vi "Substitute Actor.vi"(10 "Substitute Actor in":refnum<class "Actor.lvclass">, 11 "Current ViewableActor":refnum<class "ViewableActor.lvclass">) -> (0 "error out":errorcluster, 2 "Substitute Actor out":refnum<class "Actor.lvclass">)   [LabVIEW 2020, in "ViewableActor.lvlib" / "ViewableActor.lvclass"]
doc: "(<B>Filename</B>: Actor Framework.lvlib:Actor.lvclass:Substitute Actor.vi)\n\nThis method copies information from the <b>Current Actor</b> to the <b>Substitute Actor</b>, including the to-self and the to-caller queue references. The purpose of this function is to allow an actor to define a method that replaces itself with another actor, useful for implementing a State Pattern Actor. Child classes should override this method to copy any additional fields that they need from the current to the substitute.\n\nThis method may return error code 678010: Illegal substitution. Overrides of this method may choose to return this error if the new actor is not one that is an appropriate substitute for the current actor, for whatever standards of \"appropriate\" are chosen for the current actor. If returning an error, override VIs should return the unmodified <b>Current Actor</b> as <b>Substitute Actor out</b>."
uses:
  ViewableActor.lvclass
  C:/Program Files (x86)/National Instruments/LabVIEW 2020/vi.lib/ActorFramework/Actor/Actor.lvclass
  <vilib>/ActorFramework/Actor/Actor.lvclass
  ViewableActor.lvclass/ViewableActor.ctl
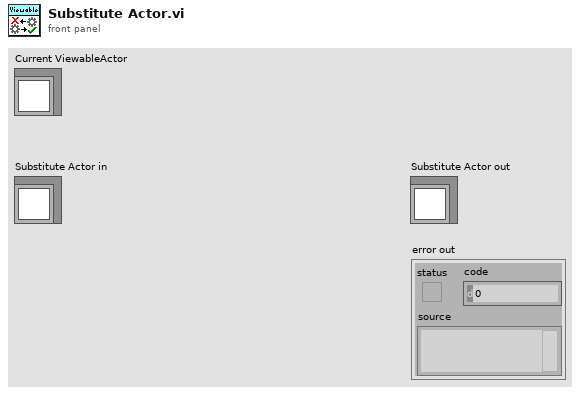
[diagram p1: front panel]
types:
  T1 = typedef "LVRectTypeDef.ctl" = cluster{"Left":i16, "Top":i16, "Right":i16, "Bottom":i16}
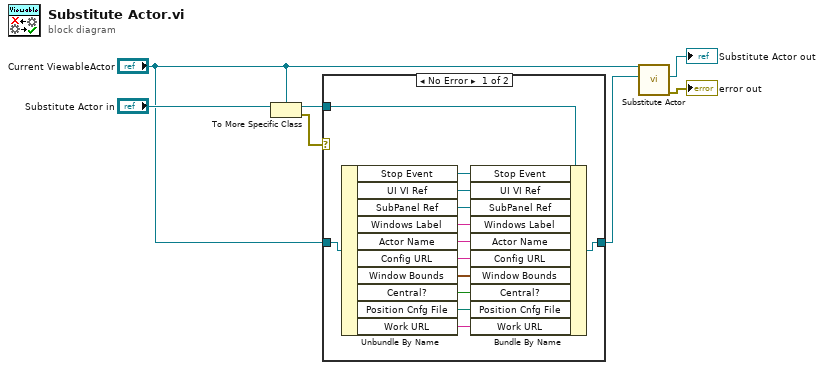
[diagram p0: block diagram]
diagram:
  n1 = To More Specific Class(target class="Current ViewableActor", reference="Substitute Actor in") -> (specific class reference=w4:refnum<class "ViewableActor.lvclass">, error out=w1:errorcluster)  [unwired: 1 in]
  n2 = case shown="No Error" w1 {
    tunnel: w4 -> [w20 _]
    tunnel: "Current ViewableActor" -> [w19 w21]
    tunnel: [w18 w21] -> w2
    frame No Error {
      n3 = Unbundle By Name(w19) -> ("Stop Event"=w17:refnum<user-event>, "UI VI Ref"=w16:refnum<vi>, "SubPanel Ref"=w15:refnum<vi>, "Windows Label"=w14:string, "Actor Name"=w13:string, "Config URL"=w12:string, "Window Bounds"=w11:T1, "Central?"=w10:bool, "Position Cnfg File"=w9:path, "Work URL"=w8:string)
      n4 = Bundle By Name(cluster=w20, "Stop Event"=w17, "UI VI Ref"=w16, "SubPanel Ref"=w15, "Windows Label"=w14, "Actor Name"=w13, "Config URL"=w12, "Window Bounds"=w11, "Central?"=w10, "Position Cnfg File"=w9, "Work URL"=w8) -> (w18:refnum<class "ViewableActor.lvclass">)
    }
    frame Error {
    }
  }
  n5 = call-parent "Substitute Actor.vi"("Substitute Actor in"=w2, "Current Actor"="Current ViewableActor") -> ("error out"=→"error out":errorcluster, "Substitute Actor out"=→"Substitute Actor out":refnum<class "Actor.lvclass">)  [unwired: 8 in]
